vi "dIMU zero sensors.vi"(0 "NXT 2":T2, 2 "Port":T3 items=["Port 1", "Port 2", "Port 3", "Port 4"], 9 "Maximum Range":enum8{"2g", "4g", "8g"}(ring), 11 "Gyro Scale":u8(ring)=16 items=["250 deg/s"=0, "500 deg/s"=16, "2000 deg/s"=32]) -> (4 "NXT":T2={"Hardware"="NXT", "Flattened String"=""}, 8 "Sensor Offsets":T1)   [LabVIEW 2010]
uses:
  <vilib>/NXT/Block Support/NXT_InputPort.ctl
  <vilib>/NXT/Subs/LVHSConnector.ctl
  dIMU_Accel_gs.vi
  dIMU_Gyro_rads.vi
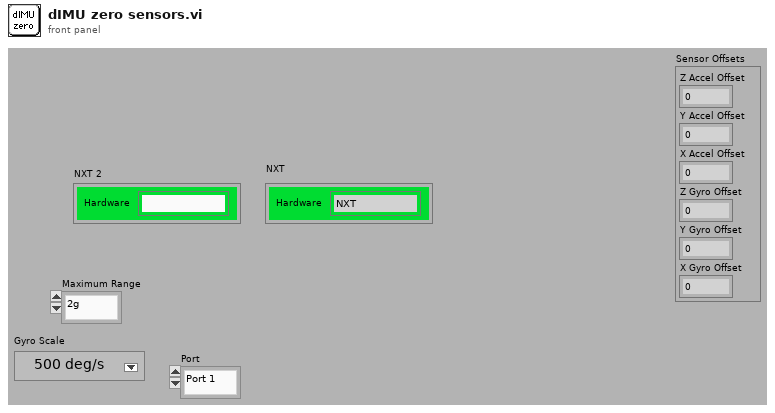
[diagram p1: front panel]
types:
  T1 = cluster{"Z Accel Offset":dbl, "Y Accel Offset":dbl, "X Accel Offset":dbl, "Z Gyro Offset":dbl, "Y Gyro Offset":dbl, "X Gyro Offset":dbl}
  T2 = typedef "LVHSConnector.ctl" = cluster{"Hardware":string, "Flattened String":string}
  T3 = typedef "NXT_InputPort.ctl" = u8
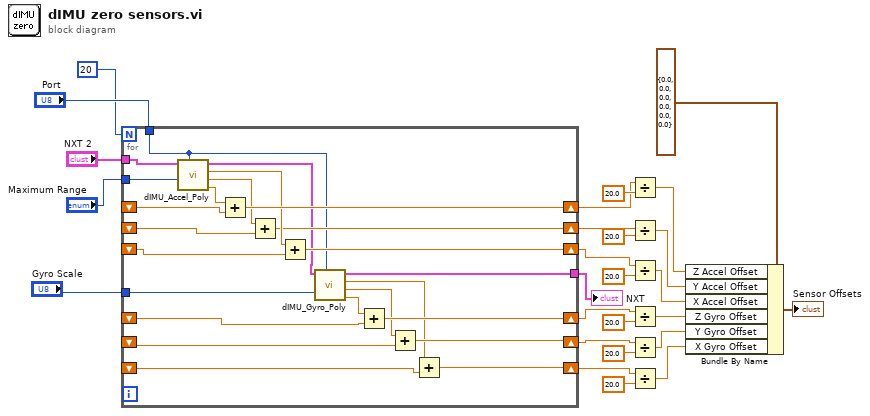
[diagram p0: block diagram]
diagram:
  n1 = for {
    N: 20 -> [_]
    tunnel: "Maximum Range" -> [w28]
    tunnel: "NXT 2" -> [w32]
    tunnel: "Port" -> [w27]
    shift-right: [w43] -> w5
    shift-left: _ -> [w42]
    shift-right: [w44] -> w6
    shift-left: _ -> [w45]
    shift-right: [w48] -> w7
    shift-left: _ -> [w49]
    shift-right: [w34] -> w2
    shift-left: _ -> [w33]
    shift-right: [w37] -> w3
    shift-left: _ -> [w36]
    shift-right: [w40] -> w4
    shift-left: _ -> [w39]
    tunnel: "Gyro Scale" -> [w29]
    tunnel: [w30] -> w1
    n2 = call-poly "dIMU_Accel_Poly.vi"("Port"=w27, "Maximum Range"=w28, "NXT"=w32) -> ("Z Accel (g)"=w50:dbl, "Y Accel (g)"=w47:dbl, "X Accel (g)"=w46:dbl, "NXT"=w31:T2)  [unwired: 5 in]
    n3 = Add(x=w50, y=w49) -> (x+y=w48:dbl)
    n4 = Add(x=w47, y=w45) -> (x+y=w44:dbl)
    n5 = Add(x=w46, y=w42) -> (x+y=w43:dbl)
    n6 = call-poly "dIMU_Gyro_Poly.vi"("Port"=w27, "Gyro Scale"=w29, "NXT"=w31) -> ("Z Gyro (rad/s"=w41:dbl, "Y Gyro (rad/s)"=w38:dbl, "X Gyro (rad/s)"=w35:dbl, "NXT"=w30:T2)  [unwired: 5 in]
    n7 = Add(x=w41, y=w39) -> (x+y=w40:dbl)
    n8 = Add(x=w38, y=w36) -> (x+y=w37:dbl)
    n9 = Add(x=w35, y=w33) -> (x+y=w34:dbl)
  }
  "NXT" <- w1
  n10 = Divide(x=w7, y=20.0) -> (x/y=w15:dbl)
  n11 = Divide(x=w6, y=20.0) -> (x/y=w14:dbl)
  n12 = Divide(x=w5, y=20.0) -> (x/y=w13:dbl)
  n13 = Divide(x=w4, y=20.0) -> (x/y=w12:dbl)
  n14 = Divide(x=w3, y=20.0) -> (x/y=w11:dbl)
  n15 = Divide(x=w2, y=20.0) -> (x/y=w10:dbl)
  n16 = Bundle By Name(cluster=T1 {"Z Accel Offset"=0.0, "Y Accel Offset"=0.0, "X Accel Offset"=0.0, "Z Gyro Offset"=0.0, "Y Gyro Offset"=0.0, "X Gyro Offset"=0.0} ("Sensor Offsets"), "Z Accel Offset"=w15, "Y Accel Offset"=w14, "X Accel Offset"=w13, "Z Gyro Offset"=w12, "Y Gyro Offset"=w11, "X Gyro Offset"=w10) -> (→"Sensor Offsets":T1)
